vi "Adquirir Imagen.vi"(8 "error in (no error)":errorcluster, 11 "Camara in":refnum<class "Camara.lvclass">) -> (0 "error out":errorcluster, 2 "Imagen":T1, 3 "Camara out":refnum<class "Camara.lvclass">)   [LabVIEW 2020, in "Camara.lvclass"]
uses:
  Camara.lvclass
  <vilib>/vision/Image Controls.llb/IMAQ Image.ctl
  <vilib>/Utility/error.llb/Error Cluster From Error Code.vi
  <vilib>/ErrorRing/Error Ring.xnode
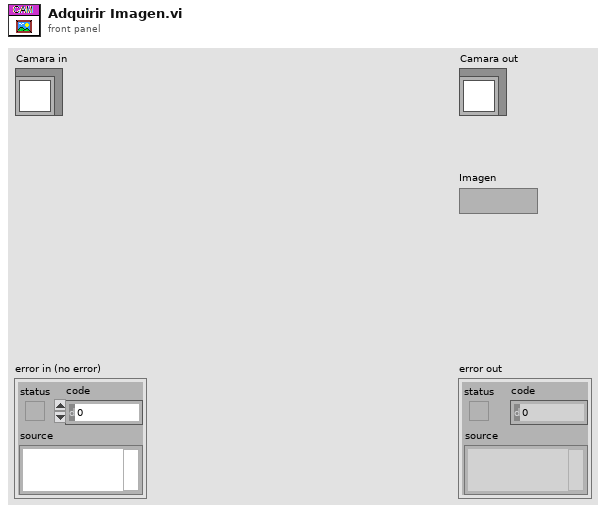
[diagram p1: front panel]
types:
  T1 = typedef "IMAQ Image.ctl" = refnum<image>
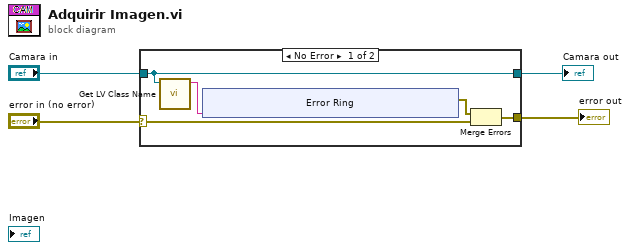
[diagram p0: block diagram]
diagram:
  n1 = case shown="No Error" "error in (no error)" {
    selector: "error in (no error)" -> [w9 w18]
    tunnel: [w8 w18] -> w3
    tunnel: [w6 w17] -> w1
    tunnel: "Camara in" -> [w6 w17]
    frame No Error {
      n2 = call <vilib>:"Get LV Class Name.vi"("object"=w6) -> ("class name"=w5:string)  [unwired: 9 in, 1 out]
      n3 = xnode "Error Ring"("parameter 0"=w5) -> ("error out"=w7:errorcluster)
      n4 = Merge Errors(w7, w9) -> (w8:errorcluster)
    }
    frame Error {
    }
  }
  "error out" <- w3
  "Camara out" <- w1
